vi "4000_Append_checksum.vi"(1 "ADAM command":string) -> (0 "ADAM string to send":string)   [LabVIEW 2010]
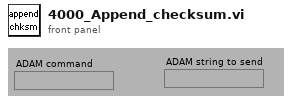
[diagram p1: front panel]
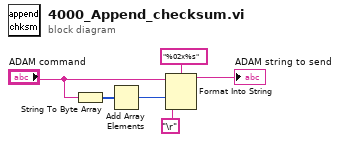
[diagram p0: block diagram]
diagram:
  n1 = String To Byte Array(string="ADAM command") -> (unsigned byte array=w1:u8[])
  n2 = Add Array Elements(numeric array=w1) -> (sum=w2:u8)
  n3 = Format Into String(format string="%02x%s", initial string="ADAM command", w2, "\r") -> (resulting string=→"ADAM string to send":string)  [unwired: 1 in, 1 out]
